vi "LEBITVacuum.PubMon&EnableEvents.vi"(0 "i ref in":refnum<vi>, 2 "i attribute in":T4={"setValuePLC"=[], "nickNames"=[], "setValuePLCServiceID"=[], "monValuePLC"=[], "SetValueServiceID"=[], "MonValueServiceID"=[], "SetValue"=[], "AllPLCValues"=[], "CondSpecial2DArray"=[], "CondSpecialIndex"=[], "ReasonForLocking"="", "ReasonForLockingID"=0, "enableValuePLC"=[], "OverwriteCloseSafetyPLC"=[], "OverwriteOpenSafetyPLC"=[], "OverwriteCloseSafetyPLCServiceID"=[], "OverwriteOpenSafetyPLCServiceID"=[], "MKS Address Array"=[], "MKS MeasurementServiceID"=[], "MKS Measurement"=[], "CRYO Measurement"=[], "CRYO MeasurementServiceID"=[], "Special"=[], "Start Date"="", "MKS VISA resource"="COM13", "CRYO VISA resource"="COM13"}, 5 "error in":errorcluster) -> (14 "i ref out":refnum<vi>, 16 "i attribute out":T4={"setValuePLC"=[], "nickNames"=[], "setValuePLCServiceID"=[], "monValuePLC"=[], "SetValueServiceID"=[], "MonValueServiceID"=[], "SetValue"=[], "AllPLCValues"=[], "CondSpecial2DArray"=[], "CondSpecialIndex"=[], "ReasonForLocking"="", "ReasonForLockingID"=0, "enableValuePLC"=[], "OverwriteCloseSafetyPLC"=[], "OverwriteOpenSafetyPLC"=[], "OverwriteCloseSafetyPLCServiceID"=[], "OverwriteOpenSafetyPLCServiceID"=[], "MKS Address Array"=[], "MKS MeasurementServiceID"=[], "MKS Measurement"=[], "CRYO Measurement"=[], "CRYO MeasurementServiceID"=[], "Special"=[], "Start Date"="", "MKS VISA resource"="COM13", "CRYO VISA resource"="COM13"}, 19 "error out":errorcluster)   [LabVIEW 2014, in "LEBITVacuum.lvlib"]
uses:
  LEBITVacuum.lvlib
  LEBITVacuum.i attribute.ctl
  CS_Core/BaseProcess/BaseProcess.event definition.ctl
  CS_Core/CAEObj/CAEObj.event definition.ctl
  CS_Core/BaseProcess/BaseProcess.descriptor string definition.ctl
  CS_Core/BaseProcess/BaseProcess.lvlib
  CS_Core/CAEObj/CAEObj.lvlib
panel:
  in  "event definition":T1
  in  "CAEEvtDef":T2
  in  "CAEEvtDef":T2
  in  "event definition":T1
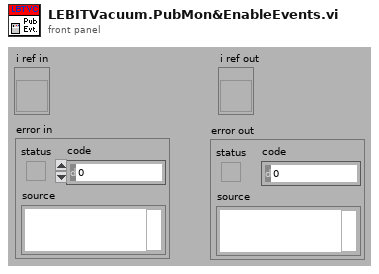
[diagram p1: front panel]
types:
  T1 = typedef "BaseProcess.lvlib/BaseProcess.event definition.ctl" = cluster{"CAEEvtDef":T2, "Data Descriptor":T3}
  T2 = typedef "CAEObj.lvlib/CAEObj.event definition.ctl" = cluster{"URL":string, "enable":bool, "ignoreResID":bool}
  T3 = typedef "BaseProcess.lvlib/BaseProcess.descriptor string definition.ctl" = string
  T4 = typedef "LEBITVacuum.lvlib/LEBITVacuum.i attribute.ctl" = cluster{"setValuePLC":string[], "nickNames":string[], "setValuePLCServiceID":i32[], "monValuePLC":string[], "SetValueServiceID":i32[], "MonValueServiceID":i32[], "SetValue":i16[], "AllPLCValues":string[], "CondSpecial2DArray":string[][], "CondSpecialIndex":i32[], "ReasonForLocking":string, "ReasonForLockingID":i32, "enableValuePLC":string[], "OverwriteCloseSafetyPLC":string[], "OverwriteOpenSafetyPLC":string[], "OverwriteCloseSafetyPLCServiceID":i32[], "OverwriteOpenSafetyPLCServiceID":i32[], "MKS Address Array":i32[][], "MKS MeasurementServiceID":i32[], "MKS Measurement":string[], "CRYO Measurement":string[][], "CRYO MeasurementServiceID":i32[], "Special":string[], "Start Date":string, "MKS VISA resource":refnum<visa-resource-name>, "CRYO VISA resource":refnum<visa-resource-name>}
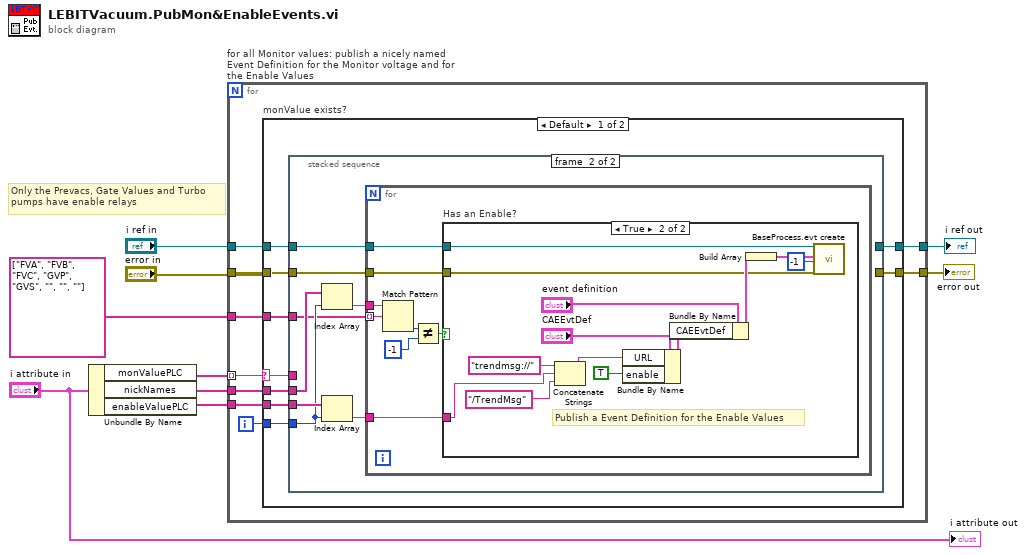
[diagram p0: block diagram]
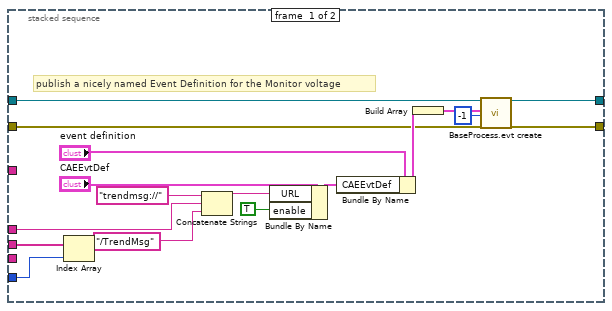
[diagram p2: hidden frame]
diagram:
  # "Only the Prevacs, Gate Values and Turbo\npumps have enable relays"
  n1 = Unbundle By Name("i attribute in") -> ("monValuePLC"=w3:string[], "nickNames"=w6:string[], "enableValuePLC"=w2:string[])
  n2 = for "for all Monitor values: publish a nicely named Event Definition for the Monitor voltage and for the Enable Values" {
    tunnel: w3 -> [w18] mode=indexing
    tunnel: w6 -> [w17]
    tunnel: "i ref in" -> [w15]
    tunnel: "error in" -> [w14]
    tunnel: [w13] -> w8
    tunnel: [w12] -> w7
    tunnel: w2 -> [w11]
    tunnel: string[] ["FVA", "FVB", "FVC", "GVP", "GVS", "", "", ""] -> [w10]
    i -> [w16]
    n3 = case "monValue exists?" shown="Default" w18 {
      selector: w18 -> [w21 _]
      tunnel: w17 -> [w27 _]
      tunnel: w16 -> [w26 _]
      tunnel: w15 -> [w25 w75]
      tunnel: w14 -> [w24 w74]
      tunnel: [w22 w74] -> w13
      tunnel: [w23 w75] -> w12
      tunnel: w11 -> [w20 _]
      tunnel: w10 -> [w19 _]
      frame Default {
        n4 = stacked-sequence {
          tunnel: w27 -> [w29 w48]
          tunnel: w26 -> [w44 w47]
          tunnel: w25 -> [w39 w52]
          tunnel: w24 -> [w38 w51]
          tunnel: [w37 _] -> w23
          tunnel: [w36 _] -> w22
          tunnel: w21 -> [w28 _]
          tunnel: w20 -> [_ w50]
          tunnel: w19 -> [_ w46]
          frame #0 {
            # "publish a nicely named Event Definition for the Monitor voltage"
            n5 = Index Array(array=w29, index=w44) -> ()  [unwired: 1 out]
            n6 = Concatenate Strings("trendmsg://" ("string"), w28, "/TrendMsg" ("string")) -> (w33:string)
            n7 = Bundle By Name(cluster="CAEEvtDef", "URL"=w33, "enable"=TRUE) -> (w41:T2)
            n8 = Bundle By Name(cluster="event definition", "CAEEvtDef"=w41) -> (w42:T1)
            n9 = Build Array(w42) -> (w43:T1[])
            n10 = call "BaseProcess.evt create.vi"("i ref in"=w39, "newEvents"=w43, "ms timeout (10000)"=-1, "error in (no error)"=w38) -> ("i ref out"=w37:refnum<vi>, "error out"=w36:errorcluster)  [unwired: 12 in, 2 out]
          }
          frame #1 {
            n11 = Index Array(array=w48, index=w47) -> (element=w45:string)
            n12 = Index Array(array=w50, index=w47) -> (element=w49:string)
            n13 = for {
              tunnel: w52 -> [w60]
              tunnel: w51 -> [w59]
              tunnel: w49 -> [w58]
              tunnel: w46 -> [w56] mode=indexing
              tunnel: w45 -> [w57]
              n14 = Match Pattern(string=w57, regular expression=w56) -> (offset past match=w55:i32)  [unwired: 1 in, 3 out]
              n15 = Not Equal?(x=w55, y=-1) -> (x != y?=w54:bool)
              n16 = case "Has an Enable?" shown="True" w54 {
                tunnel: w60 -> [_ w69]
                tunnel: w59 -> [_ w68]
                tunnel: w58 -> [_ w61]
                frame False {
                }
                frame True {
                  # "Publish a Event Definition for the Enable Values"
                  n17 = Concatenate Strings("trendmsg://" ("string"), w61, "/TrendMsg" ("string")) -> (w65:string)
                  n18 = Bundle By Name(cluster="CAEEvtDef", "URL"=w65, "enable"=TRUE) -> (w71:T2)
                  n19 = Bundle By Name(cluster="event definition", "CAEEvtDef"=w71) -> (w72:T1)
                  n20 = Build Array(w72) -> (w73:T1[])
                  n21 = call "BaseProcess.evt create.vi"("i ref in"=w69, "newEvents"=w73, "ms timeout (10000)"=-1, "error in (no error)"=w68) -> ()  [unwired: 12 in, 4 out]
                }
              }
            }
          }
        }
      }
      frame "" {
      }
    }
  }
  "error out" <- w8
  "i ref out" <- w7
  "i attribute out" <- "i attribute in"
